vi "S2C_Shared_Proc_TranslateParameters.vi"(8 "Error In":errorcluster, 11 "Data":variant) -> (0 "Error Out":errorcluster, 3 "JSON Cluster":string)   [LabVIEW 2024]
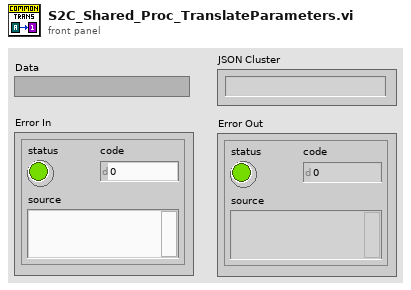
[diagram p1: front panel]
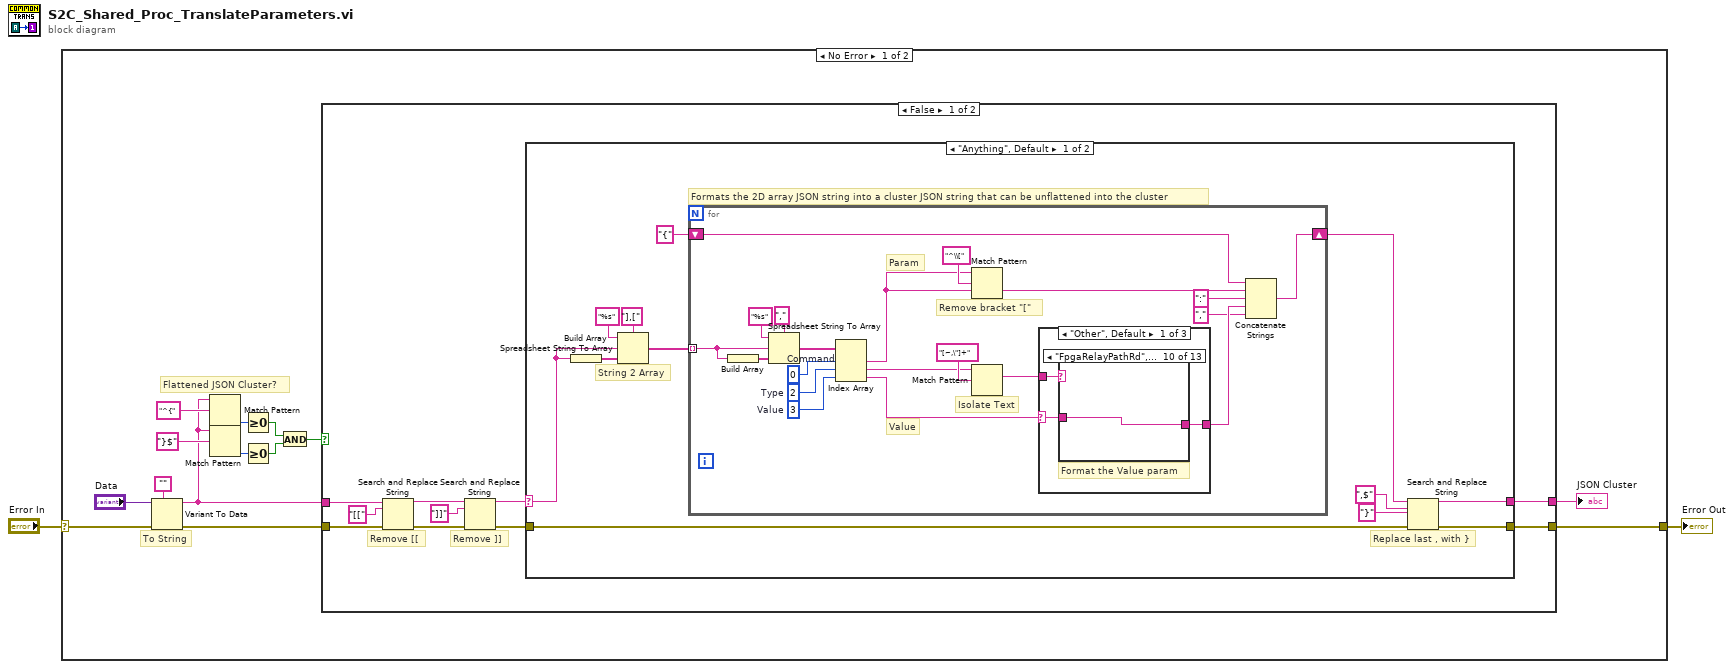
[diagram p0: block diagram]
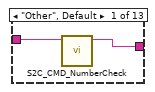
[diagram p2: hidden frame]
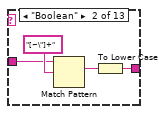
[diagram p3: hidden frame]
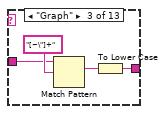
[diagram p4: hidden frame]
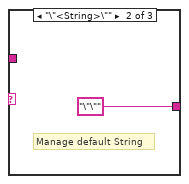
[diagram p14: hidden frame]
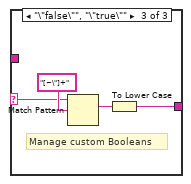
[diagram p15: hidden frame]
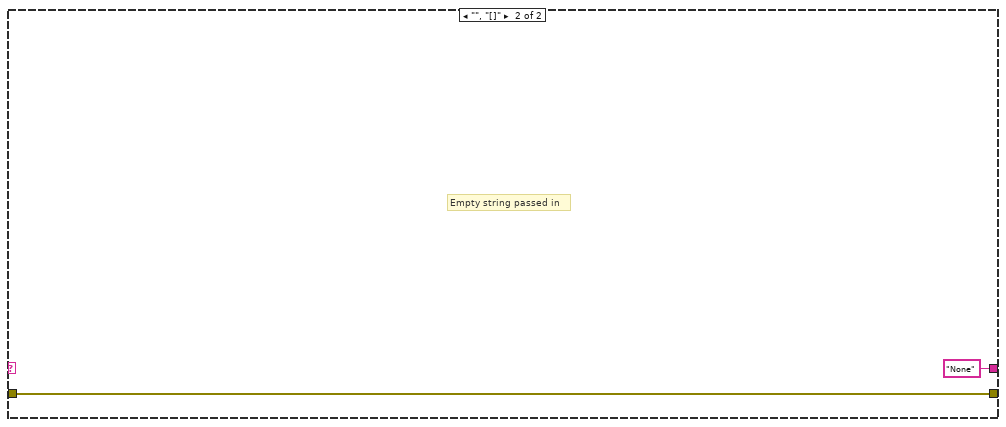
[diagram p16: hidden frame]
diagram:
  n1 = case shown="No Error" "Error In" {
    selector: "Error In" -> [w13 w89]
    tunnel: [w15 w89] -> w1
    frame No Error {
      # "Flattened JSON Cluster?"
      # "To String"
      n2 = Variant To Data(error in=w13, type="", Variant="Data") -> (data=w4:string, error out=w12:errorcluster)
      n3 = Match Pattern(string=w4, regular expression="^{") -> (offset past match=w10:i32)  [unwired: 1 in, 3 out]
      n4 = Match Pattern(string=w4, regular expression="}$") -> (offset past match=w9:i32)  [unwired: 1 in, 3 out]
      n5 = Greater Or Equal To 0?(x=w10) -> (x >= 0?=w6:bool)
      n6 = Greater Or Equal To 0?(x=w9) -> (x >= 0?=w5:bool)
      n7 = And(x=w6, y=w5) -> (x .and. y?=w3:bool)
      n8 = case shown="False" w3 {
        tunnel: [w24 w88] -> w16
        tunnel: [w22 w87] -> w15
        tunnel: w12 -> [w19 w87]
        tunnel: w4 -> [w17 w88]
        frame False {
          # "Remove ]]"
          # "Remove [["
          n9 = Search and Replace String(input string=w17, search string="[[", error in=w19) -> (result string=w20:string, error out=w23:errorcluster)  [unwired: 5 in, 2 out]
          n10 = Search and Replace String(input string=w20, search string="]]") -> (result string=w18:string)  [unwired: 6 in, 3 out]
          n11 = case shown="\"Anything\", Default" w18 {
            selector: w18 -> [w26 _]
            tunnel: [w29 "None" ("result string")] -> w24
            tunnel: w23 -> [w28 w86]
            tunnel: [w27 w86] -> w22
            frame "Anything", Default {
              # "Formats the 2D array JSON string into a cluster JSON string that can be unflattened into the cluster"
              # "Replace last , with }"
              # "String 2 Array"
              n12 = Build Array(w26) -> (w35:string[])
              n13 = Spreadsheet String To Array(delimiter (Tab)="],[", format string="%s", spreadsheet string=w26, array type (2D Dbl)=w35) -> (array=w34:string[])
              n14 = for {
                tunnel: w34 -> [w41] mode=indexing
                shift-right: [w50] -> w33
                shift-left: "{" -> [w51]
                w42 = 3  # Value
                w43 = 2  # Type
                w44 = 0  # Command
                # "Remove bracket \"[\""
                # "Isolate Text"
                # "Value"
                # "Param"
                n15 = Build Array(w41) -> (w46:string[])
                n16 = Spreadsheet String To Array(delimiter (Tab)=",", format string="%s", spreadsheet string=w41, array type (2D Dbl)=w46) -> (array=w45:string[])
                n17 = Index Array(array=w45, index #1=w44, index #2=w43, index #3=w42) -> (element #1=w39:string, element #2=w40:string, element #3=w38:string)
                n18 = Match Pattern(string=w39, regular expression="^\\[") -> ()  [unwired: 1 in, 4 out]
                n19 = Match Pattern(string=w40, regular expression="[~,\"]+") -> (match substring=w54:string)  [unwired: 1 in, 3 out]
                n20 = case shown="\"Other\", Default" w38 {
                  selector: w38 -> [w57 _ w82]
                  tunnel: w54 -> [w59 _ _]
                  tunnel: [w58 "\"\"" w81] -> w53
                  frame "Other", Default {
                    # "Format the Value param"
                    n21 = case shown="\"FpgaRelayPathRd\", \"FpgaRelayPathWr\"" w59 {
                      tunnel: w57 -> [w61 w64 w68 w70 w71 w72 w73 w74 w75 w76 w77 w78 w79]
                      tunnel: [w60 w62 w66 w70 w71 w72 w73 w74 w75 w76 w77 w78 w79] -> w58
                      frame "Other", Default {
                        n22 = call "S2C_CMD_NumberCheck.vi"("String In"=w61) -> ("String Out"=w60:string)  [unwired: 8 in, 2 out]
                      }
                      frame "Boolean" {
                        n23 = Match Pattern(string=w64, regular expression="[~\"]+") -> (match substring=w63:string)  [unwired: 1 in, 3 out]
                        n24 = To Lower Case(string=w63) -> (all lower case string=w62:string)
                      }
                      frame "Graph" {
                        n25 = Match Pattern(string=w68, regular expression="[~\"]+") -> (match substring=w67:string)  [unwired: 1 in, 3 out]
                        n26 = To Lower Case(string=w67) -> (all lower case string=w66:string)
                      }
                      frame "String" {
                      }
                      frame "FpgaAudio" {
                      }
                      frame "FpgaHandSwitchRd", "FpgaHandSwitchWr" {
                      }
                      frame "FpgaHomerRd", "FpgaHomerWr" {
                      }
                      frame "FpgaLxfRd", "FpgaLxfWr" {
                      }
                      frame "FpgaPalletRd", "FpgaSmokeEvacRd" {
                      }
                      frame "FpgaRelayPathRd", "FpgaRelayPathWr" {
                      }
                      frame "FpgaRemRd", "FpgaRemWr" {
                      }
                      frame "FpgaReserved", "FpgaTriverse" {
                      }
                      frame "FpgaVlacRd", "FpgaVlacWr" {
                      }
                    }
                  }
                  frame "\"<String>\"" {
                    # "Manage default String"
                  }
                  frame "\"false\"", "\"true\"" {
                    # "Manage custom Booleans"
                    n27 = Match Pattern(string=w82, regular expression="[~\"]+") -> (match substring=w83:string)  [unwired: 1 in, 3 out]
                    n28 = To Lower Case(string=w83) -> (all lower case string=w81:string)
                  }
                }
                n29 = Concatenate Strings(w51, w39, ":" ("string"), w53, "," ("string")) -> (w50:string)
              }
              n30 = Search and Replace String(input string=w33, search string=",$", replace string="}" ("replace string (\"\")"), error in=w28) -> (result string=w29:string, error out=w27:errorcluster)  [unwired: 4 in, 2 out]
            }
            frame "", "[]" {
              # "Empty string passed in"
            }
          }
        }
        frame True {
          # "Braces at beginning and end of flattened string indicate it is already a cluster, no need to translate from 2D array."
        }
      }
      "JSON Cluster" <- w16
    }
    frame Error {
    }
  }
  "Error Out" <- w1
